vi "LVClass_DataServer SetBoolean.vi"(0 "DataServer in":refnum<class "DataServer.lvclass">, 5 "name":string, 7 "Value":bool, 11 "error in (no error)":errorcluster) -> (4 "DataServer out":refnum<class "DataServer.lvclass">, 15 "error out":errorcluster)   [LabVIEW 2020, in "DataServer.lvclass"]
doc: "Set the slopes to be send by TCP connection.\n\n--------------------------------------------------------------------------------\n\n<B>serverIn </B> : Server object.\n<B>serverOut </B> : Server object.\n<B>hasoslopes </B> : HasoSlopes object.\n<B>ErrorIn </B> : Error\n<B>ErrorOut </B> : Error\n\n--------------------------------------------------------------------------------"
uses:
  DataServer.lvclass
  DataServer.lvclass/DataServer.ctl
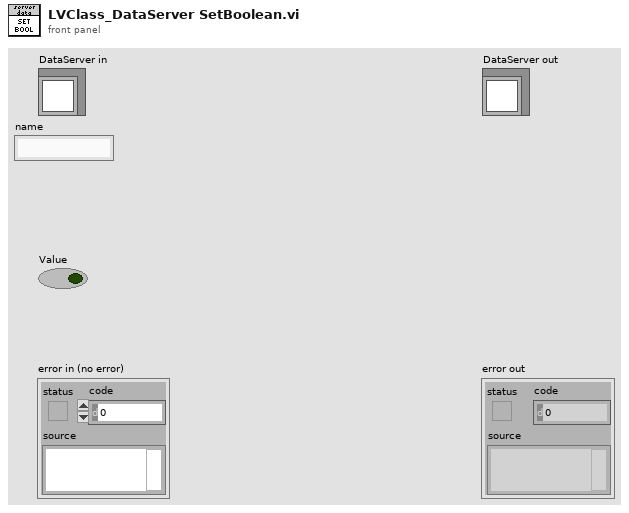
[diagram p1: front panel]
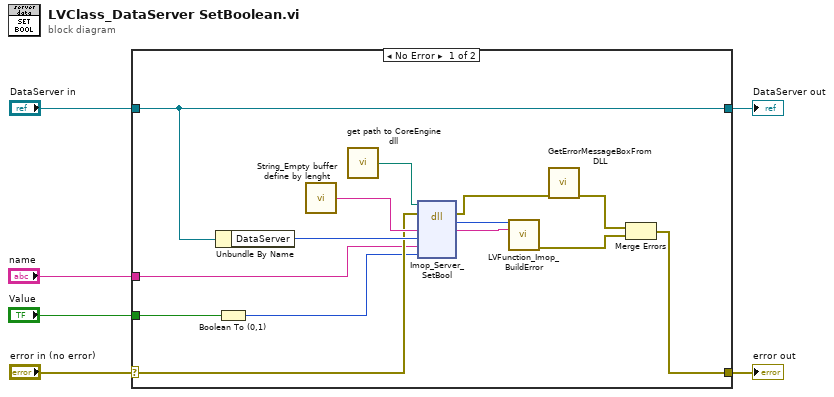
[diagram p0: block diagram]
diagram:
  n1 = case shown="No Error" "error in (no error)" {
    selector: "error in (no error)" -> [w11 w22]
    tunnel: [w10 w22] -> w5
    tunnel: [w12 w21] -> w3
    tunnel: "DataServer in" -> [w12 w21]
    tunnel: "Value" -> [w7 _]
    tunnel: "name" -> [w9 _]
    frame No Error {
      n2 = Unbundle By Name(w12) -> ("DataServer"=w18:i32)
      n3 = Boolean To (0,1)(Boolean=w7) -> (0, 1=w8:i16)
      n4 = call "String_Empty buffer define by lenght.vi"() -> ("Empty buffer"=w15:string)  [unwired: 1 in]
      n5 = call "get path to CoreEngine dll.vi"() -> ("path to c_interface_vc100.dll"=w16:path)  [unwired: 12 in, 3 out]
      n6 = dll-call lib="D:/soft/HASO_v3/SVN_trunk/ImOpCoreEngine4_LV2011/DLLs/c_interface_vc100.dll" fn="Imop_Server_SetBool"(path in=w16, error in=w11, "message"=w15, "server"=w18, "name"=w9, "data"=w8) -> (error out=w17:errorcluster, "return type"=w13:i32, "message"=w14:string)  [unwired: 4 in, 1 out]
      n7 = call "LVFunction_Imop_BuildError.vi"("code"=w13, "String to Prepend to source (\"\")"=w14) -> ("error out"=w20:errorcluster)  [unwired: 13 in]
      n8 = call "GetErrorMessageBoxFromDLL.vi"("error IN"=w17) -> ("error OUT"=w19:errorcluster)  [unwired: 10 in]
      n9 = Merge Errors(w19, w20) -> (w10:errorcluster)
    }
    frame Error {
    }
  }
  "error out" <- w5
  "DataServer out" <- w3
